vi "Drive_Hardware_Globals.vi"() -> ()   [LabVIEW 2020]
panel:
  in  "Back_Right_CANcoder":string="Back_Right_CANcoder"
  in  "Back_Left_CANcoder":string="Back_Left_CANcoder"
  in  "Front_Left_CANcoder":string="Front_Left_CANcoder"
  in  "Front_Right_CANcoder":string="Front_Right_CANcoder"
  in  "Swerve_IMU":string="Swerve_IMU"
  in  "Swerve_Drive_Front_Right_Ref":string="Swerve_Drive_Front_Right_Ref"
  in  "Swerve_Azimuth_Front_Right_Ref":string="Swerve_Azimuth_Front_Right_Ref"
  in  "Swerve_Drive_Back_Right_Ref":string="Swerve_Drive_Back_Right_Ref"
  in  "Swerve_Azimuth_Back_Right_Ref":string="Swerve_Azimuth_Back_Right_Ref"
  in  "Swerve_Drive_Back_Left_Ref":string="Swerve_Drive_Back_Left_Ref"
  in  "Swerve_Azimuth_Back_Left_Ref":string="Swerve_Azimuth_Back_Left_Ref"
  in  "Swerve_Drive_Front_Left_Ref":string="Swerve_Drive_Front_Left_Ref"
  in  "Swerve_Azimuth_Front_Left_Ref":string="Swerve_Azimuth_Front_Left_Ref"
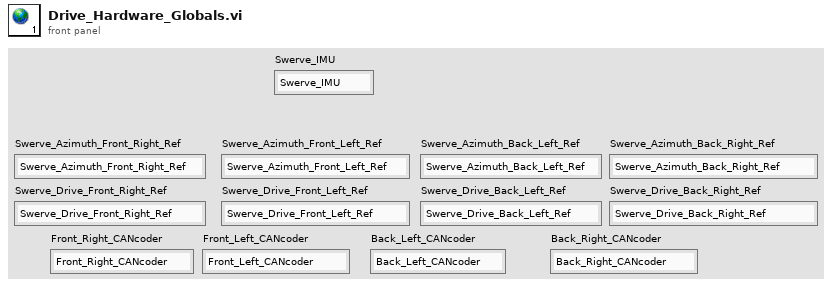
[diagram p1: front panel]
diagram:
